vi "Get Clusters String Name.vi"(11 "error in":errorcluster) -> (4 "control names out":string[](array[string]), 6 "array size":i32, 15 "error out":errorcluster)   [LabVIEW 2021, in "Converter Reusables.lvlib"]
uses:
  Converter Reusables.lvlib
  TypeDefs/Dictionary States.ctl
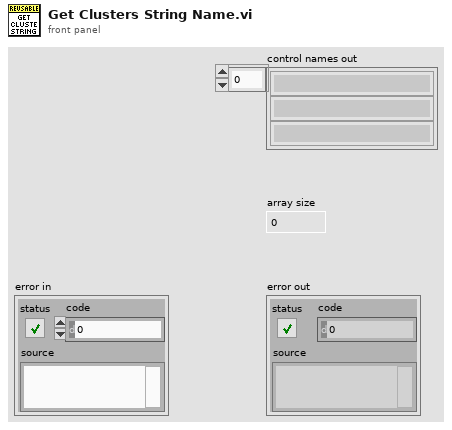
[diagram p1: front panel]
types:
  T1 = typedef "Converter Reusables.lvlib/Dictionary States.ctl" = enum16{"Set", "Get", "Delete", "Delete All"}
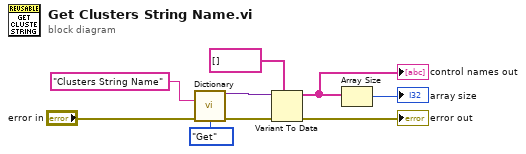
[diagram p0: block diagram]
diagram:
  n1 = call "Dictionary.vi"("key"="Clusters String Name" ("Key"), "error in"="error in", "dict states"=Dictionary_States."Get" ("Dict States")) -> ("variant out"=w8:variant, "error out"=w3:errorcluster)  [unwired: 11 in]
  n2 = Variant To Data(error in=w3, type=string[] [], Variant=w8) -> (data=w5:string[], error out=→"error out":errorcluster)
  "control names out" <- w5
  n3 = Array Size(array=w5) -> (size(s)=→"array size":i32)
